vi "Cull and Group.vi"(6 "Line Border":cluster{"Top":dbl, "Bottom":dbl}={"Top"=6.0, "Bottom"=1.0}, 9 "Score Cutoff":dbl=3.0, 10 "Sorted Data":dbl[][](array[numeric])) -> (0 "Rect":T1, 1 "Line":T1, 2 "Score":dbl, 3 "Center":cluster{"X":dbl, "Y":dbl})   [LabVIEW 2016]
doc: "Examine the particle measurements to find the most likely pair that make up the target. This mostly compares the edges of the bounding boxes. It then returns information about the overall target, notably the rectangle sourrounding the particles, the vertical line that bisects the target, and the center of the top particle."
panel:
  out "Grouping Scores":T2(array[cluster])
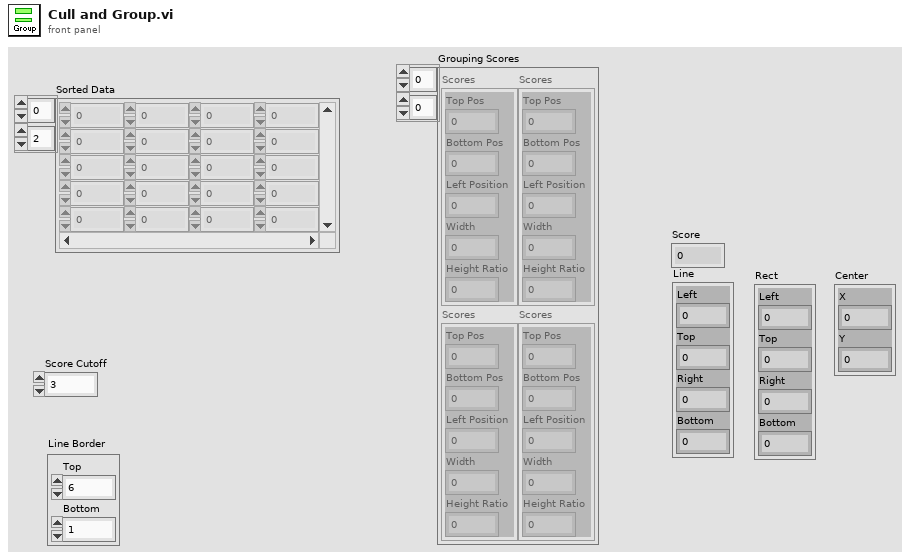
[diagram p1: front panel]
types:
  T1 = cluster{"Left":dbl, "Top":dbl, "Right":dbl, "Bottom":dbl}
  T2 = cluster{"Top Pos":dbl, "Bottom Pos":dbl, "Left Position":dbl, "Width":dbl, "Height Ratio":dbl}[][]
  T3 = cluster{"Top Position":dbl, "Bottom Position":dbl, "Left Gap":dbl, "Width":dbl, "Height Ratio":dbl}
  T4 = cluster{"Left":dbl, "Numeric":dbl, "Right":dbl, "Numeric":dbl}
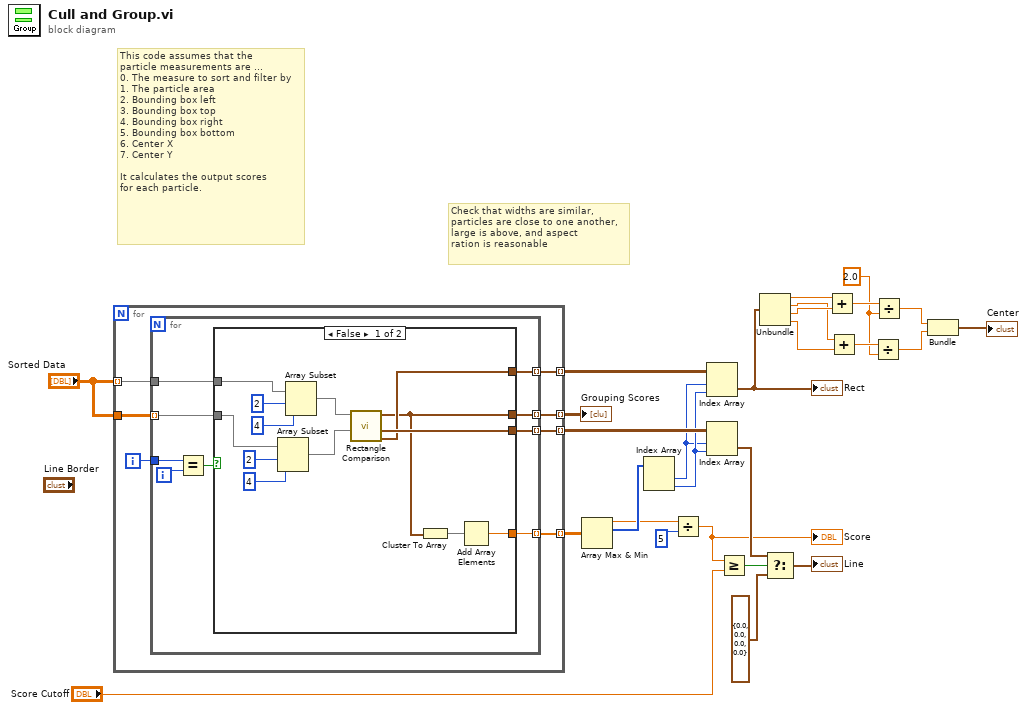
[diagram p0: block diagram]
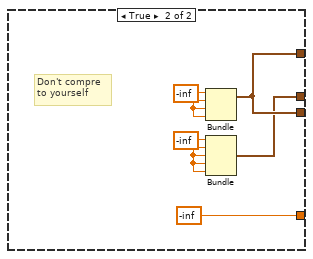
[diagram p2: hidden frame]
diagram:
  w4 = 2.0 ("y")
  # "Check that widths are similar,\nparticles are close to one another,\nlarge is above, and aspect\nration is reasonable"
  # "This code assumes that the\nparticle measurements are ...\n0. The measure to sort and filter by\n1. The particle area\n2. Bounding box left\n3. Bounding box top\n4. Bounding box right\n5. Bounding box bottom\n6. Center X\n7. Center Y\n\nIt calculates the output scores\nfor each particle."
  n1 = for {
    tunnel: "Sorted Data" -> [w34] mode=indexing
    tunnel: "Sorted Data" -> [w33]
    tunnel: [w32] -> w27 mode=indexing
    tunnel: [w30] -> w26 mode=indexing
    tunnel: [w29] -> w23 mode=indexing
    tunnel: [w28] -> w19 mode=indexing
    i -> [w31]
    n2 = for {
      tunnel: w34 -> [w43]
      tunnel: w33 -> [w41] mode=indexing
      tunnel: [w40] -> w32 mode=indexing
      tunnel: w31 -> [w39]
      tunnel: [w37] -> w30 mode=indexing
      tunnel: [w36] -> w29 mode=indexing
      tunnel: [w35] -> w28 mode=indexing
      i -> [w38]
      n3 = Equal?(x=w39, y=w38) -> (x = y?=w42:bool)
      n4 = case shown="False" w42 {
        tunnel: w43 -> [w54 _]
        tunnel: w41 -> [w51 _]
        tunnel: [w44 w57] -> w40
        tunnel: [w49 -inf] -> w37
        tunnel: [w46 w60] -> w36
        tunnel: [w45 w60] -> w35
        frame False {
          n5 = Array Subset(array=w51, index=2, length=4) -> (w47:dbl[])
          n6 = Array Subset(array=w54, index=2, length=4) -> (w48:dbl[])
          n7 = call "Rectangle Comparison.vi"("Second"=w47, "First"=w48) -> ("Rect"=w45:T1, "Line"=w46:T1, "Scores"=w44:T3)  [unwired: 7 in]
          n8 = Cluster To Array(cluster=w44) -> (array=w50:dbl[])
          n9 = Add Array Elements(numeric array=w50) -> (sum=w49:dbl)
        }
        frame True {
          w58 = -inf
          w59 = -inf
          # "Don't compre\nto yourself"
          n10 = Bundle(w59, w59, w59, w59) -> (w60:cluster{dbl, dbl, dbl, dbl})  [unwired: 1 in]
          n11 = Bundle(w58, w58, w58, w58, w58) -> (w57:cluster{dbl, dbl, dbl, dbl, dbl})  [unwired: 1 in]
        }
      }
    }
  }
  "Grouping Scores" <- w27
  n12 = Array Max & Min(array=w26) -> (max value=w14:dbl, max index (indices)=w15:i32[])  [unwired: 2 out]
  n13 = Index Array(array=w15) -> (element #1=w16:i32, element #2=w18:i32)  [unwired: 2 in]
  n14 = Divide(x=w14, y=5 ("length")) -> (x/y=w13:dbl)
  "Score" <- w13
  n15 = Index Array(array=w19, index (row)=w16, index (col)=w18) -> (element=w11:T1)
  "Rect" <- w11
  n16 = Index Array(array=w23, index (row)=w16, index (col)=w18) -> (element=w22:T1)
  n17 = Greater Or Equal?(x=w13, y="Score Cutoff") -> (x >= y?=w25:bool)
  n18 = Unbundle(w11) -> ("Left"=w10:dbl, "Top"=w7:dbl, "Right"=w9:dbl, "Bottom"=w6:dbl)
  n19 = Select(t=w22, s=w25, f=cluster{dbl, "Numeric":dbl, dbl, "Numeric":dbl} {0.0, "Numeric"=0.0, 0.0, "Numeric"=0.0}) -> (s? t:f=→"Line":T4)
  n20 = Add(x=w10, y=w9) -> (x+y=w8:dbl)
  n21 = Add(x=w7, y=w6) -> (x+y=w5:dbl)
  n22 = Divide(x=w5, y=w4) -> (x/y=w2:dbl)
  n23 = Divide(x=w8, y=w4) -> (x/y=w3:dbl)
  n24 = Bundle(w3, w2) -> (→"Center":cluster{dbl, dbl})  [unwired: 1 in]
